vi "Read Image.vi"(8 "Error In":errorcluster, 11 "File Path":path) -> (0 "Error Out":errorcluster, 2 "Image":T1(plugin-control), 3 "Image Pixels (I16)":u8[][](array[numeric]))   [LabVIEW 2018, in "Image Management.lvlib"]
uses:
  Image Management.lvlib
  Action.ctl
  <vilib>/vision/Image Controls.llb/IMAQ Image.ctl
panel:
  # "Make this Image control!!!"
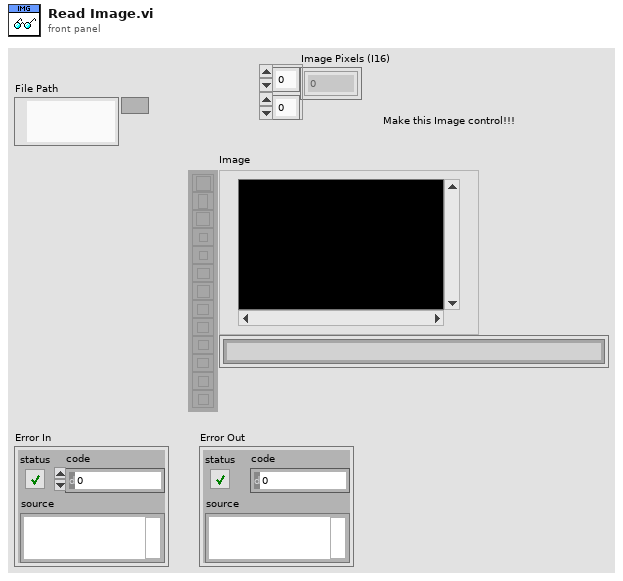
[diagram p1: front panel]
types:
  T1 = typedef "IMAQ Image.ctl" = refnum<image>
  T2 = cluster{"Image Pixels (U8)":u8[][], "Image Out":T1}
  T3 = typedef "Image Management.lvlib/Action.ctl" = enum16{"Init", "Find Linespaces", "Get Image Size (pixels)", "Close"}
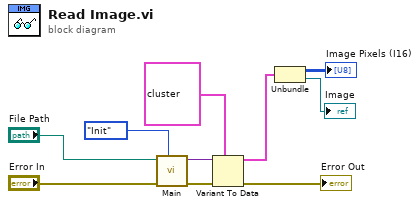
[diagram p0: block diagram]
diagram:
  n1 = call "Main.vi"("Action"=Action."Init", "Error In"="Error In", "File Path to Load"="File Path") -> ("Error Out"=w9:errorcluster, "Output"=w8:variant)  [unwired: 7 in]
  n2 = Variant To Data(error in=w9, type=T2 {"Image Pixels (U8)"=[], "Image Out"=refnum} ("output cluster"), Variant=w8) -> (data=w3:T2, error out=→"Error Out":errorcluster)
  n3 = Unbundle(w3) -> ("Image Pixels (U8)"=→"Image Pixels (I16)":u8[][], "Image Out"=→"Image":T1)
